vi "triggeID.vi"() -> ()   [LabVIEW 2017]
panel:
  out "diff":i32[][](array[numeric])
  out "错误输出":errorcluster
  out "end":i32[][](array[numeric])
  out "counter":i32[][](array[numeric])
  out "begin":i32[][](array[numeric])
  out "analysis":i32[][](array[numeric])
  out "求和":i32
  out "trigger number":u64=23048 format="%x"
  out "substring 2":string
  out "PAD NO":u64
  out "TDC_ID":u64=6
  out "Middle ID":u64=2
  out "x与y？":u64
  out "substring 3":string
  out "data 3":string="Z"
  in  "dat file (use dialog)":path=path "G:/tdc/2017/test_20250325_114227.dat"
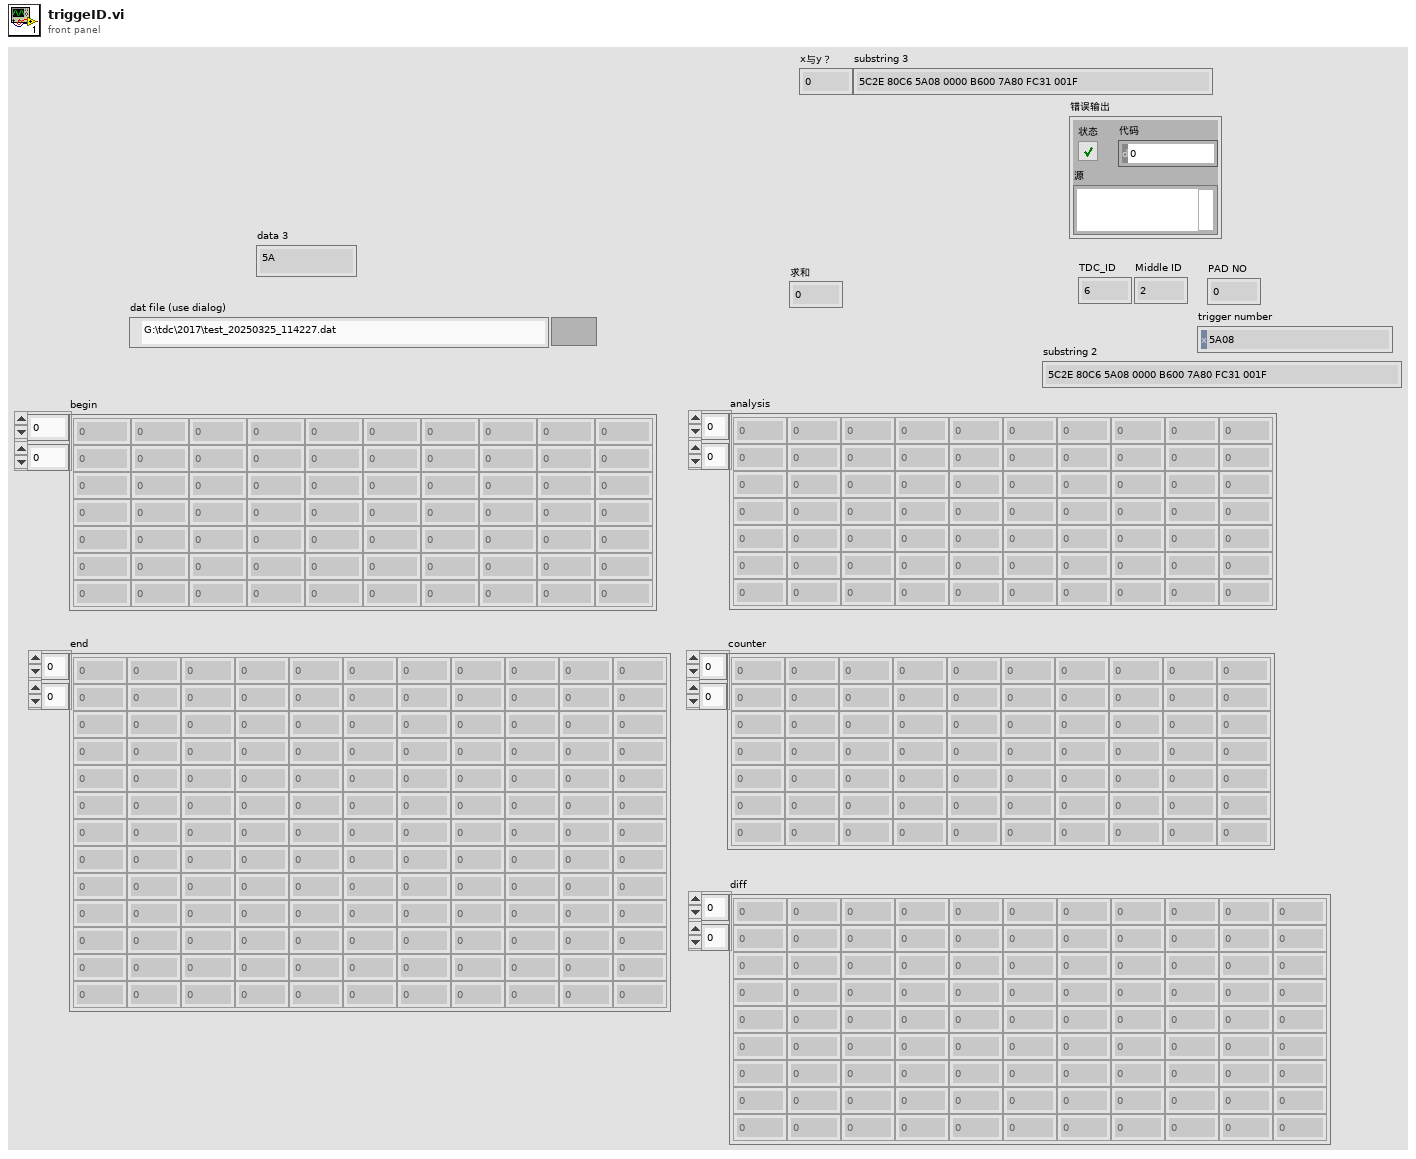
[diagram p1: front panel]
types:
  T1 = enum16{"open", "replace", "create", "open or create", "replace or create", "replace or create with confirmation"}
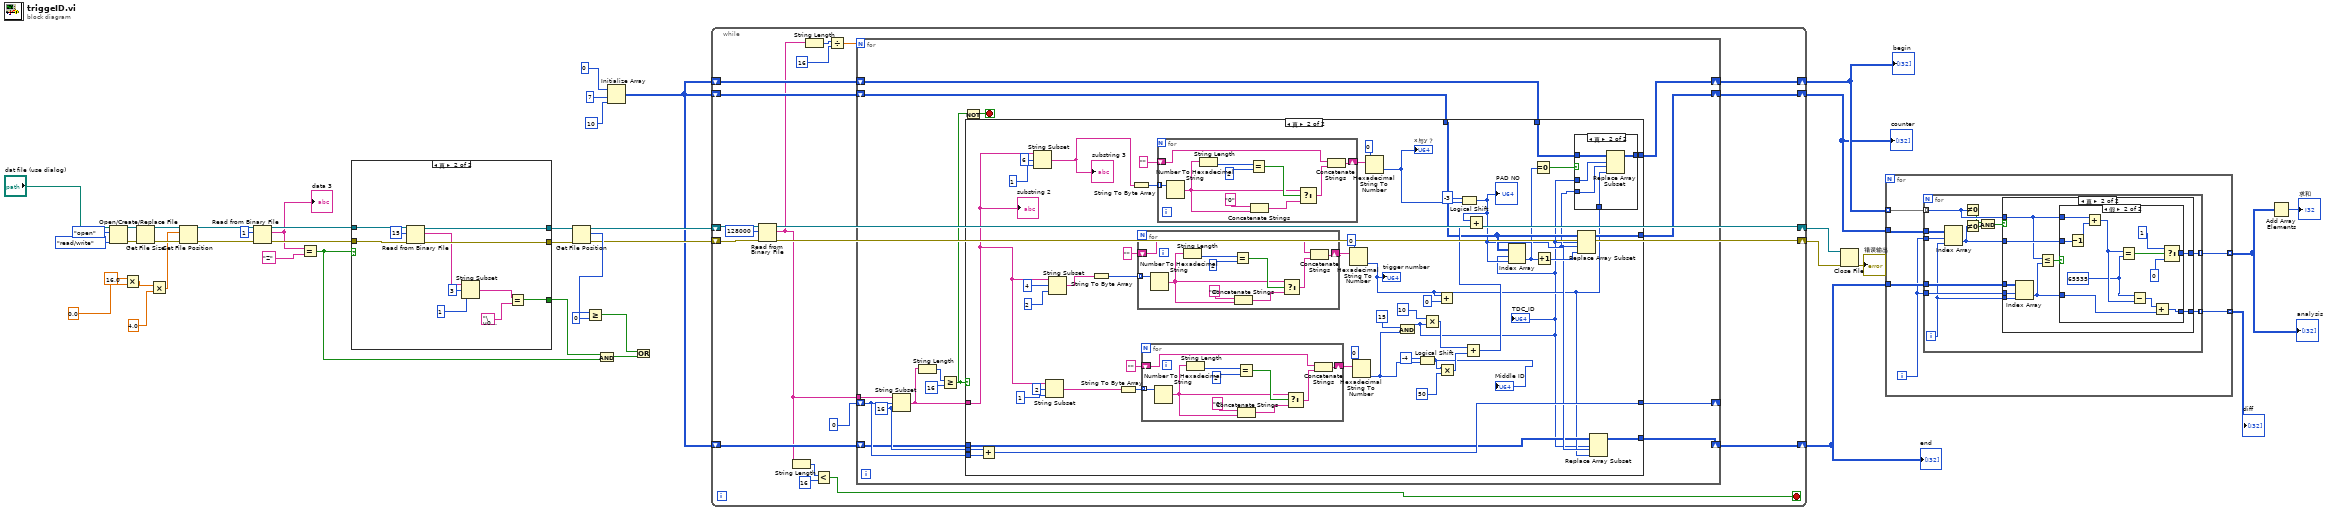
[diagram p0: block diagram]
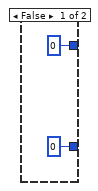
[diagram p2: hidden frame]
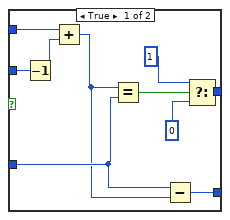
[diagram p3: hidden frame]
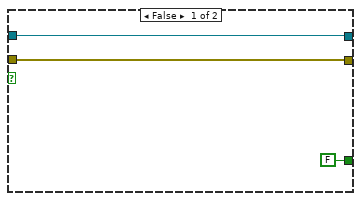
[diagram p6: hidden frame]
diagram:
  n1 = Open/Create/Replace File(file path (use dialog)="dat file (use dialog)", operation (0:open)=T1."open", access (0:read/write)=enum16{"read/write", "read-only", "write-only"}."read/write") -> (refnum out=w42:refnum<file>, error out=w39:errorcluster)  [unwired: 3 in, 1 out]
  n2 = Multiply(x=16.0, y=0.0) -> (x*y=w33:dbl)
  n3 = Get File Size(file=w42, error in=w39) -> (refnum out=w37:refnum<file>, 0:w36:errorcluster)  [unwired: 1 out]
  n4 = Multiply(x=w33, y=4.0) -> (x*y=w31:dbl)
  n5 = Set File Position(offset (in bytes) (0)=w31, refnum=w37, error in=w36) -> (refnum out=w18:refnum<file>, error out=w17:errorcluster)  [unwired: 1 in]
  n6 = Read from Binary File(8:w17, 10:1 ("count (1)"), 11:w18) -> (0:w27:errorcluster, 2:w25:string, 3:w28:refnum<file>)  [unwired: 3 in, 1 out]
  "data 3" <- w25
  n7 = Equal?(x=w25, y="Z") -> (x = y?=w22:bool)
  n8 = case shown="真" w22 {
    tunnel: w28 -> [w45 w56]
    tunnel: w27 -> [w44 w55]
    tunnel: [w45 w53] -> w26
    tunnel: [w44 w52] -> w21
    tunnel: [FALSE w46] -> w23
    frame False {
    }
    frame True {
      n9 = Read from Binary File(8:w55, 10:15 ("count (1)"), 11:w56) -> (0:w52:errorcluster, 2:w49:string, 3:w53:refnum<file>)  [unwired: 3 in, 1 out]
      n10 = String Subset(string=w49, offset (0)=3, length (rest)=1 ("length (rest)")) -> (substring=w48:string)
      n11 = Equal?(x=w48, y="\u0000") -> (x = y?=w46:bool)
    }
  }
  n12 = Get File Position(4:w21, 7:w26) -> (0:w14:errorcluster, 2:w20:i64, 3:w15:refnum<file>)
  n13 = Greater Or Equal?(x=w20, y=i64 0) -> (x >= y?=w19:bool)
  n14 = Compound Arithmetic op=AND(w23, w22) -> (w24:bool)
  n15 = Initialize Array(0 ("元素"), 7 ("维数大小"), 10 ("维数大小")) -> (w10:i32[][])
  n16 = Or(x=w19, y=w24) -> ()  [unwired: 1 out]
  n17 = while {
    shift-right: [w67] -> w8
    shift-left: w10 -> [w68]
    shift-right: [w65] -> w9
    shift-left: w10 -> [w66]
    shift-right: [w63] -> w7
    shift-left: w10 -> [w64]
    shift-right: [w62] -> w4
    shift-left: w15 -> [w75]
    shift-right: [w61] -> w3
    shift-left: w14 -> [w74]
    stop <- w57 stop-if-true
    n18 = Read from Binary File(8:w74, 10:128000 ("总数(1)"), 11:w75) -> (0:w61:errorcluster, 2:w58:string, 3:w62:refnum<file>)  [unwired: 3 in, 1 out]
    n19 = String Length(string=w58) -> (length=w59:i32)
    n20 = String Length(string=w58) -> (length=w71:i32)
    n21 = Less?(x=w59, y=16 ("length (rest)")) -> (x < y?=w57:bool)
    n22 = Divide(x=w71, y=16 ("length (rest)")) -> (x/y=w70:dbl)
    n23 = for {
      N: w70 -> [_]
      tunnel: w58 -> [w90]
      shift-right: [w88] -> w67
      shift-left: w68 -> [w89]
      shift-right: [w80] -> _
      shift-left: 0 -> [w81]
      shift-right: [w78] -> w65
      shift-left: w66 -> [w79]
      shift-right: [w76] -> w63
      shift-left: w64 -> [w77]
      stop <- w83 stop-if-true
      w82 = 16 ("length (rest)")
      n24 = String Subset(string=w90, offset (0)=w81, length (rest)=w82) -> (substring=w87:string)
      n25 = String Length(string=w87) -> (length=w86:i32)
      n26 = Greater Or Equal?(x=w86, y=16 ("length (rest)")) -> (x >= y?=w84:bool)
      n27 = Not(x=w84) -> (.not. x?=w83:bool)
      n28 = case shown="真" w84 {
        tunnel: w87 -> [_ w128]
        tunnel: w89 -> [w94 w106]
        tunnel: [w94 w127] -> w88
        tunnel: w81 -> [w93 w126]
        tunnel: w82 -> [_ w125]
        tunnel: [w93 w124] -> w80
        tunnel: w79 -> [w92 w103]
        tunnel: [w92 w101] -> w78
        tunnel: w77 -> [w91 w99]
        tunnel: [w91 w98] -> w76
        frame False {
        }
        frame True {
          n29 = Add(x=w125, y=w126) -> (x+y=w124:i32)
          n30 = String Subset(string=w128, offset (0)=6, length (rest)=1 ("length (rest)")) -> (substring=w108:string)
          "substring 3" <- w108
          n31 = String Subset(string=w128, offset (0)=2, length (rest)=1 ("length (rest)")) -> (substring=w119:string)
          n32 = String Subset(string=w128, offset (0)=4, length (rest)=2 ("length (rest)")) -> (substring=w135:string)
          n33 = String To Byte Array(string=w135) -> (unsigned byte array=w137:u8[])
          n34 = String To Byte Array(string=w119) -> (unsigned byte array=w122:u8[])
          n35 = String To Byte Array(string=w108) -> (unsigned byte array=w131:u8[])
          n36 = for {
            shift-right: [w178] -> w138
            shift-left: "" ("format string") -> [w175]
            tunnel: w137 -> [w179] mode=indexing
            n37 = Number To Hexadecimal String(2:w179) -> (0:w171:string)  [unwired: 1 in]
            n38 = String Length(string=w171) -> (length=w177:i32)
            n39 = Equal?(x=w177, y=2) -> (x = y?=w174:bool)
            n40 = Concatenate Strings("0" ("format string"), w171) -> (w173:string)
            n41 = Select(t=w171, s=w174, f=w173) -> (s? t:f=w170:string)
            n42 = Concatenate Strings(w175, w170) -> (w178:string)
          }
          n43 = for {
            shift-right: [w158] -> w121
            shift-left: "" ("format string") -> [w155]
            tunnel: w122 -> [w159] mode=indexing
            n44 = Number To Hexadecimal String(2:w159) -> (0:w151:string)  [unwired: 1 in]
            n45 = String Length(string=w151) -> (length=w157:i32)
            n46 = Equal?(x=w157, y=2) -> (x = y?=w154:bool)
            n47 = Concatenate Strings("0" ("format string"), w151) -> (w153:string)
            n48 = Select(t=w151, s=w154, f=w153) -> (s? t:f=w150:string)
            n49 = Concatenate Strings(w155, w150) -> (w158:string)
          }
          n50 = for {
            shift-right: [w168] -> w130
            shift-left: "" ("format string") -> [w165]
            tunnel: w131 -> [w169] mode=indexing
            n51 = Number To Hexadecimal String(2:w169) -> (0:w161:string)  [unwired: 1 in]
            n52 = String Length(string=w161) -> (length=w167:i32)
            n53 = Equal?(x=w167, y=2) -> (x = y?=w164:bool)
            n54 = Concatenate Strings("0" ("format string"), w161) -> (w163:string)
            n55 = Select(t=w161, s=w164, f=w163) -> (s? t:f=w160:string)
            n56 = Concatenate Strings(w165, w160) -> (w168:string)
          }
          n57 = Hexadecimal String To Number(string=w138, default (0uL)=u64 0 ("default (0 U32)")) -> (number=w97:u64)  [unwired: 1 in, 1 out]
          "trigger number" <- w97
          n58 = Hexadecimal String To Number(string=w121, default (0uL)=u64 0 ("default (0 U32)")) -> (number=w114:u64)  [unwired: 1 in, 1 out]
          n59 = Hexadecimal String To Number(string=w130, default (0uL)=u64 0 ("default (0 U32)")) -> (number=w107:u64)  [unwired: 1 in, 1 out]
          "x与y？" <- w107
          n60 = And(x=u64 15 ("default (0 U32)"), y=w114) -> (x .and. y?=w96:u64)
          "TDC_ID" <- w96
          n61 = Logical Shift(y=i16 -4, x=w114) -> (x << y=w95:u64)
          "Middle ID" <- w95
          n62 = Multiply(x=u64 10, y=w96) -> (x*y=w110:u64)
          n63 = Add(x=w97, y=u64 0) -> ()  [unwired: 1 out]
          n64 = Multiply(x=w95, y=u64 50 ("x")) -> (x*y=w111:u64)
          n65 = Logical Shift(y=i16 -3, x=w107) -> (x << y=w100:u64)
          "PAD NO" <- w100
          n66 = Add(x=w110, y=w111) -> (x+y=w109:u64)
          n67 = Add(x=w100, y=w109) -> ()  [unwired: 1 out]
          n68 = Index Array(array=w106, index (row)=w96, index (col)=w100) -> (element=w104:i32)
          n69 = Equal To 0?(x=w104) -> (x = 0?=w102:bool)
          n70 = Increment(x=w104) -> (x+1=w105:i32)
          n71 = case shown="真" w102 {
            tunnel: w103 -> [w144 w149]
            tunnel: w96 -> [_ w148]
            tunnel: w100 -> [_ w147]
            tunnel: w97 -> [_ w146]
            tunnel: [w144 w145] -> w101
            frame False {
            }
            frame True {
              n72 = Replace Array Subset(array=w149, new element=w146, index (row)=w148, index (col)=w147) -> (w145:i32[][])
            }
          }
          n73 = Replace Array Subset(array=w106, new element=w105, index (row)=w96, index (col)=w100) -> (w127:i32[][])
          n74 = Replace Array Subset(array=w99, new element=w97, index (row)=w96, index (col)=w100) -> (w98:i32[][])
          "substring 2" <- w128
        }
      }
    }
  }
  "begin" <- w9
  "counter" <- w8
  "end" <- w7
  n75 = Close File(refnum=w4, error in=w3) -> (error out=→"错误输出":errorcluster)  [unwired: 1 out]
  n76 = for {
    tunnel: w9 -> [w184] mode=indexing
    tunnel: w8 -> [w185]
    tunnel: w7 -> [w183]
    tunnel: [w181] -> w6 mode=indexing
    tunnel: [w180] -> w1 mode=indexing
    i -> [w182]
    n77 = for {
      tunnel: w185 -> [w197]
      tunnel: w184 -> [w190] mode=indexing
      tunnel: w182 -> [w196]
      tunnel: w183 -> [w195]
      tunnel: w182 -> [w194]
      tunnel: [w192] -> w181 mode=indexing
      tunnel: [w191] -> w180 mode=indexing
      i -> [w193]
      n78 = Index Array(array=w197, index (row)=w196, index (col)=w193) -> (element=w186:i32)
      n79 = Not Equal To 0?(x=w190) -> (x != 0?=w189:bool)
      n80 = Not Equal To 0?(x=w186) -> (x != 0?=w187:bool)
      n81 = And(x=w189, y=w187) -> (x .and. y?=w188:bool)
      n82 = case shown="真" w188 {
        tunnel: w190 -> [_ w201]
        tunnel: w186 -> [_ w208]
        tunnel: w195 -> [_ w207]
        tunnel: w194 -> [_ w206]
        tunnel: w193 -> [_ w205]
        tunnel: [0 w204] -> w192
        tunnel: [0 w203] -> w191
        frame False {
        }
        frame True {
          n83 = Index Array(array=w207, index (row)=w206, index (col)=w205) -> (element=w200:i32)
          n84 = Less Or Equal?(x=w201, y=w200) -> (x <= y?=w202:bool)
          n85 = case shown="假" w202 {
            tunnel: w201 -> [w218 w230]
            tunnel: w208 -> [w217 w229]
            tunnel: [w213 w225] -> w204
            tunnel: w200 -> [w212 w219]
            tunnel: [w210 w221] -> w203
            frame True {
              n86 = Decrement(x=w217) -> (x-1=w209:i32)
              n87 = Add(x=w218, y=w209) -> (x+y=w211:i32)
              n88 = Equal?(x=w211, y=w212) -> (x = y?=w216:bool)
              n89 = Subtract(x=w212, y=w211) -> (x-y=w210:i32)
              n90 = Select(t=1, s=w216, f=0) -> (s? t:f=w213:i32)
            }
            frame False {
              w220 = 65535
              n91 = Decrement(x=w229) -> (x-1=w223:i32)
              n92 = Add(x=w230, y=w223) -> (x+y=w224:i32)
              n93 = Equal?(x=w224, y=w220) -> (x = y?=w228:bool)
              n94 = Subtract(x=w220, y=w224) -> (x-y=w222:i32)
              n95 = Add(x=w222, y=w219) -> (x+y=w221:i32)
              n96 = Select(t=1, s=w228, f=0) -> (s? t:f=w225:i32)
            }
          }
        }
      }
    }
  }
  "analysis" <- w6
  "diff" <- w1
  n97 = Add Array Elements(numeric array=w6) -> (sum=→"求和":i32)
